vi "Launch Plot.vi"(8 "error in (no error)":errorcluster, 9 "Plot type":T1, 10 "File Path Control":path, 11 "Monitor-Pulse in":refnum<class "Monitor-Pulse.lvclass">) -> (0 "error out":errorcluster, 2 "Nested Actor's Enqueuer":refnum<class "Message Enqueuer.lvclass">, 3 "Monitor-Pulse out":refnum<class "Monitor-Pulse.lvclass">)   [LabVIEW 2015, in "Monitor-Pulse.lvclass"]
uses:
  Monitor-Pulse.lvclass
  Measure_core/Plots/Plot types.ctl
  <vilib>/ActorFramework/Message Enqueuer/Message Enqueuer.lvclass
  Monitor-Pulse.lvclass/Monitor-Pulse.ctl
  Measure_core/Measure Controller/Measure Controller.lvclass
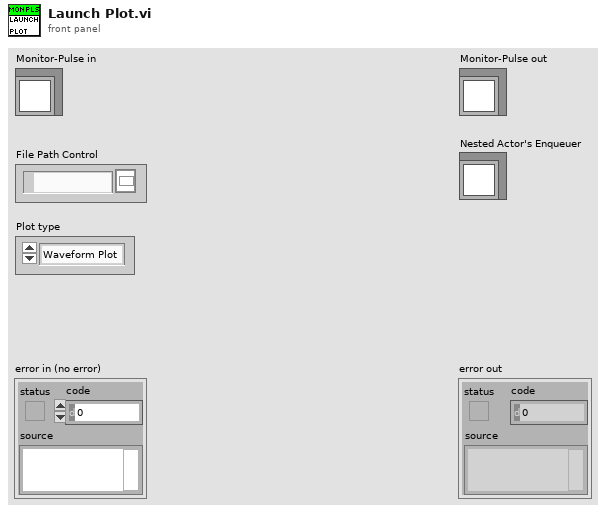
[diagram p1: front panel]
types:
  T1 = typedef "Plot types.ctl" = enum16{"Waveform Plot", "XY Plot"}
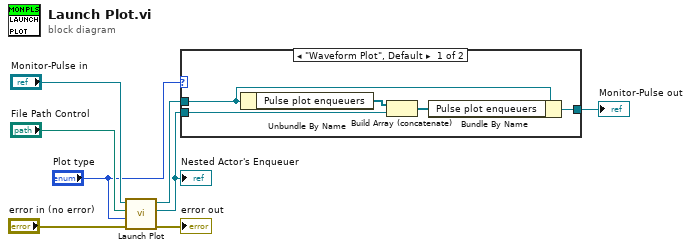
[diagram p0: block diagram]
diagram:
  n1 = call-parent "Launch Plot.vi"("error in (no error)"="error in (no error)", "Plot type"="Plot type", "File Path Control"="File Path Control", "Measure Controller in"="Monitor-Pulse in") -> ("error out"=→"error out":errorcluster, "Nested Actor's Enqueuer"=w2:refnum<class "Message Enqueuer.lvclass">, "Measure Controller out"=w3:refnum<class "Monitor-Pulse.lvclass">)  [unwired: 5 in]
  "Nested Actor's Enqueuer" <- w2
  n2 = case shown="\"Waveform Plot\", Default" "Plot type" {
    tunnel: w3 -> [w11 w14]
    tunnel: w2 -> [w12 _]
    tunnel: [w9 w14] -> w1
    frame "Waveform Plot", Default {
      n3 = Unbundle By Name(w11) -> ("Pulse plot enqueuers"=w13:refnum<class "Message Enqueuer.lvclass">[])
      n4 = Build Array (concatenate)(w13, w12) -> (w10:refnum<class "Message Enqueuer.lvclass">[])
      n5 = Bundle By Name(cluster=w11, "Pulse plot enqueuers"=w10) -> (w9:refnum<class "Monitor-Pulse.lvclass">)
    }
    frame "XY Plot" {
    }
  }
  "Monitor-Pulse out" <- w1
